vi "Append to Buffer.vi"(8 "error in":errorcluster, 10 "Channel":string, 11 "BufferLastReadsWAV in":refnum<class "BufferLastReadsWAV.lvclass">) -> (0 "error out":errorcluster, 3 "BufferLastReadsWAV out":refnum<class "BufferLastReadsWAV.lvclass">)   [LabVIEW 2024, in "BufferLastReadsWAV.lvclass"]
uses:
  BufferLastReadsWAV.lvclass
  BufferLastReadsWAV.lvclass/BufferLastReadsWAV.ctl
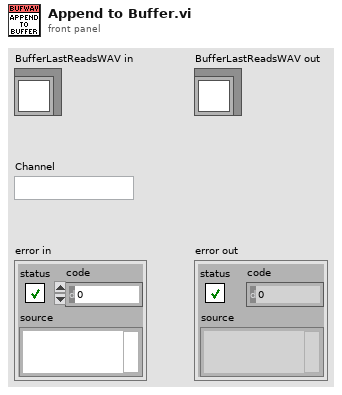
[diagram p1: front panel]
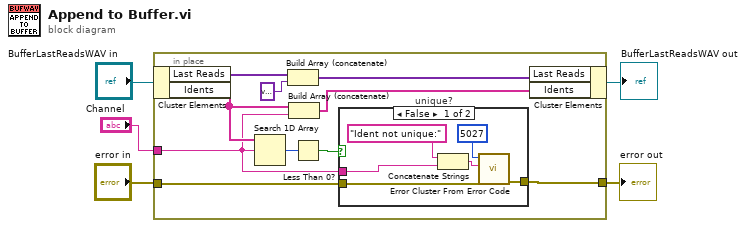
[diagram p0: block diagram]
diagram:
  n1 = in-place {
    in-place-border: [w13] -> w2
    in-place-border: "Channel" -> [w7]
    in-place-border: "error in" -> [w12]
    n2 = in-place-cluster #1("BufferLastReadsWAV in") -> ("Last Reads"=w11:variant[], "Idents"=w10:string[])
    n3 = Search 1D Array(1D array=w10, element=w7) -> (index of element=w14:i32)  [unwired: 1 in]
    n4 = Build Array (concatenate)(w11, variant) -> (w9:variant[])
    n5 = Build Array (concatenate)(w10, w7) -> (w8:string[])
    n6 = Less Than 0?(x=w14) -> (x < 0?=w15:bool)
    n7 = case "unique?" shown="False" w15 {
      tunnel: w12 -> [w21 w22]
      tunnel: [w20 w22] -> w13
      tunnel: w7 -> [w16 _]
      frame False {
        n8 = Concatenate Strings("Ident not unique:" ("string"), w16) -> (w18:string)
        n9 = call <vilib>:"Error Cluster From Error Code.vi"("error in (no error)"=w21, "error message (\"\")"=w18, "error code (0)"=5027) -> ("error out"=w20:errorcluster)  [unwired: 6 in]
      }
      frame True {
      }
    }
    n10 = in-place-cluster #1("Last Reads"=w9, "Idents"=w8) -> (→"BufferLastReadsWAV out":refnum<class "BufferLastReadsWAV.lvclass">)
  }
  "error out" <- w2
